vi "CollisionAvoidence.vi"(11 "Cluster":T1) -> (3 "output cluster":T1)   [LabVIEW 2014]
uses:
  Drive Train Metrics.ctl
  CmdFlag.ctl
  Ultrasonic Data.vi
  DriveTrainCals.vi
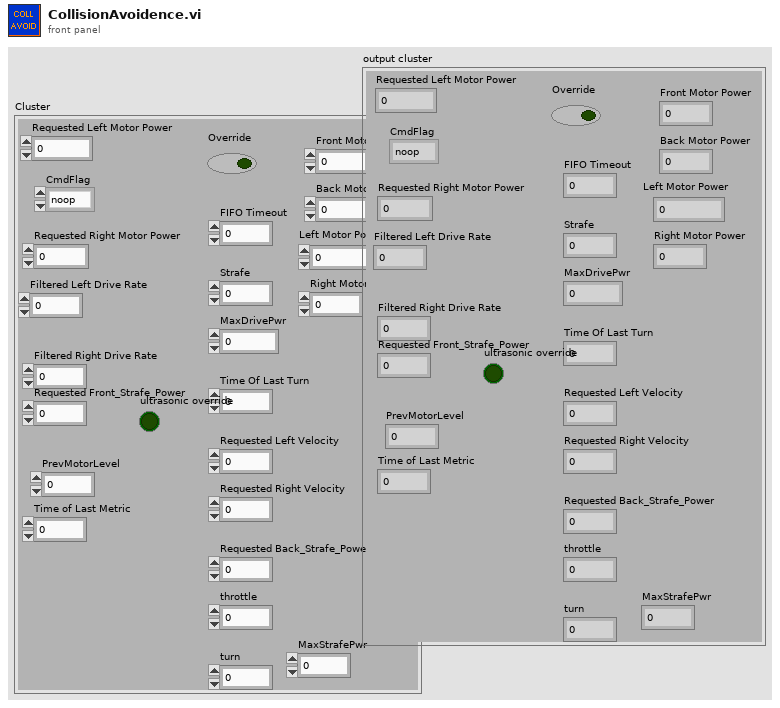
[diagram p1: front panel]
types:
  T1 = typedef "Drive Train Metrics.ctl" = cluster{"CmdFlag":T2, "Requested Right Motor Power":dbl, "Requested Left Motor Power":dbl, "Filtered Left Drive Rate":dbl, "Filtered Right Drive Rate":dbl, "Time of Last Metric":u32, "FIFO Timeout":i32, "Requested Left Velocity":dbl, "Requested Right Velocity":dbl, "throttle":dbl, "turn":dbl, "MaxDrivePwr":dbl, "Strafe":dbl, "Override":bool, "Time Of Last Turn":dbl, "Requested Front_Strafe_Power":dbl, "Requested Back_Strafe_Power":dbl, "MaxStrafePwr":dbl, "PrevMotorLevel":u8, "ultrasonic override":bool, "Left Motor Power":dbl, "Right Motor Power":dbl, "Front Motor Power":dbl, "Back Motor Power":dbl}
  T2 = typedef "CmdFlag.ctl" = enum16{"noop", "logflag", "suspend", "resume"}
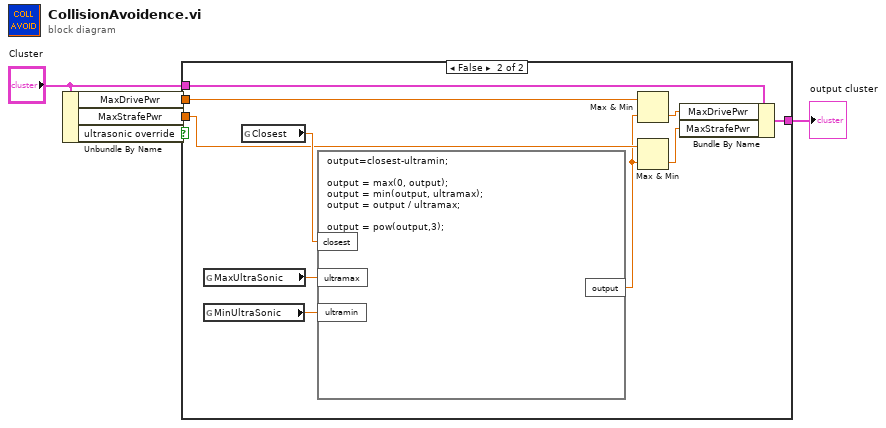
[diagram p0: block diagram]
diagram:
  n1 = Unbundle By Name("Cluster") -> ("MaxDrivePwr"=w3:dbl, "MaxStrafePwr"=w2:dbl, "ultrasonic override"=w1:bool)
  n2 = case shown="False" w1 {
    tunnel: [w6 w15] -> w5
    tunnel: "Cluster" -> [w6 w14]
    tunnel: w3 -> [_ w13]
    tunnel: w2 -> [_ w11]
    frame True {
    }
    frame False {
      n3 = global read "DriveTrainCals.vi" "MaxUltraSonic"() -> (w7:dbl)
      n4 = global read "DriveTrainCals.vi" "MinUltraSonic"() -> (w8:dbl)
      n5 = global read "Ultrasonic Data.vi" "Closest"() -> (w16:dbl)
      n6 = formula code="output=closest-ultramin;\n\noutput = max(0, output);\noutput = min(output, ultramax);\noutput = output / ultramax;\n\noutput = pow(output,3);"("closest"=w16, "ultramax"=w7, "ultramin"=w8) -> ("output"=w10:dbl)
      n7 = Max & Min(x=w13, y=w10) -> (min(x,y)=w12:dbl)  [unwired: 1 out]
      n8 = Max & Min(x=w11, y=w10) -> (min(x,y)=w9:dbl)  [unwired: 1 out]
      n9 = Bundle By Name(cluster=w14, "MaxDrivePwr"=w12, "MaxStrafePwr"=w9) -> (w15:T1)
    }
  }
  "output cluster" <- w5
